vi "Read Name.vi"(11 "ZIP Item in":refnum<class "ZIP Item.lvclass">) -> (2 "Name":string)   [LabVIEW 2019, in "ZIP.lvlib" / "ZIP Item.lvclass"]
doc: "Returns the name of the solution item.\n----\nCopyright: MGI 2017\nAuthor: Derek Trepanier"
uses:
  ZIP Item.lvclass
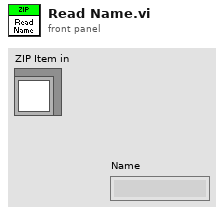
[diagram p1: front panel]
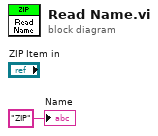
[diagram p0: block diagram]
diagram:
  "Name" <- "ZIP" ("Name")
